vi "ConvertTimes - Array.vi"(1 "GP22 results":u32[](array[numeric])) -> (0 "Array of times / s":dbl[](array[numeric]))   [LabVIEW 2013, in "GP22_TDC_Arduinoed.lvlib"]
doc: "Convert fixed point output of GP22 to time value in seconds."
uses:
  GP22_TDC_Arduinoed.lvlib
  Public/Globals.vi
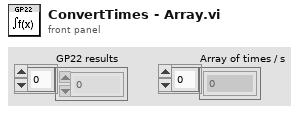
[diagram p1: front panel]
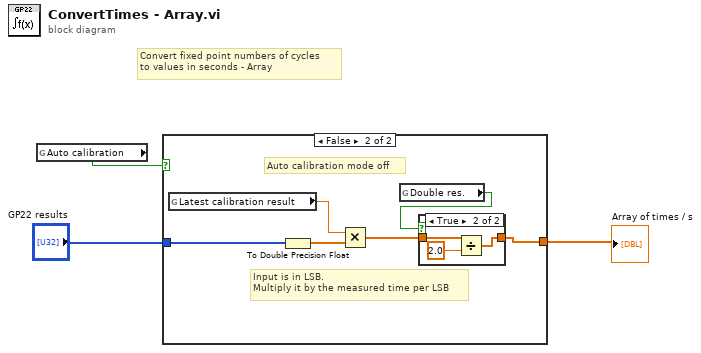
[diagram p0: block diagram]
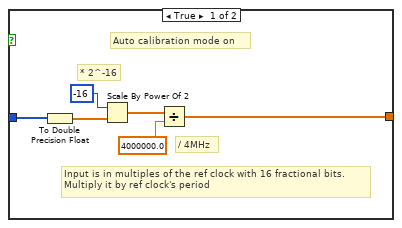
[diagram p2: hidden frame]
diagram:
  # "Convert fixed point numbers of cycles\nto values in seconds - Array"
  n1 = global read "Globals.vi" "Auto calibration"() -> (w2:bool)
  n2 = case shown="False" w2 {
    tunnel: [w7 w10] -> w1
    tunnel: "GP22 results" -> [w5 w15]
    frame True {
      # "Input is in multiples of the ref clock with 16 fractional bits.\nMultiply it by ref clock's period"
      # "Auto calibration mode on"
      # "/ 4MHz"
      # "* 2^-16"
      n3 = To Double Precision Float(number=w5) -> (double precision float=w4:dbl[])
      n4 = Scale By Power Of 2(n=i16 -16, x=w4) -> (x*2^n=w8:dbl[])
      n5 = Divide(x=w8, y=4000000.0) -> (x/y=w7:dbl[])
    }
    frame False {
      # "Input is in LSB. \nMultiply it by the measured time per LSB"
      # "Auto calibration mode off"
      n6 = global read "Globals.vi" "Latest calibration result"() -> (w13:dbl)
      n7 = To Double Precision Float(number=w15) -> (double precision float=w14:dbl[])
      n8 = Multiply(x=w13, y=w14) -> (x*y=w11:dbl[])
      n9 = global read "Globals.vi" "Double res."() -> (w12:bool)
      n10 = case shown="True" w12 {
        tunnel: w11 -> [w16 w18]
        tunnel: [w16 w17] -> w10
        frame False {
        }
        frame True {
          n11 = Divide(x=w18, y=2.0) -> (x/y=w17:dbl[])
        }
      }
    }
  }
  "Array of times / s" <- w1
